vi "Print Report.vi"(0 "report in":refnum<class "NI_HTML.lvclass">, 5 "printer name (default)":string, 9 "number of copies (1)":i32=1, 11 "error in (no error)":errorcluster) -> (4 "report out":refnum<class "NI_HTML.lvclass">, 15 "error out":errorcluster)   [LabVIEW 2020, in "NI_HTML.lvclass"]
doc: "Prints a report to a designated printer or to the default printer on the computer."
uses:
  NI_HTML.lvclass
  e:/builds/penguin/labview/branches/2020/dev/dist/vi.lib/Utility/NIReport.llb/NI_report.lvclass
  NI_ReportGenerationCore.lvlib
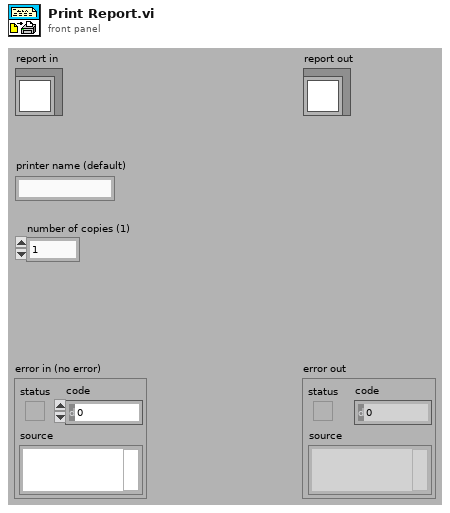
[diagram p1: front panel]
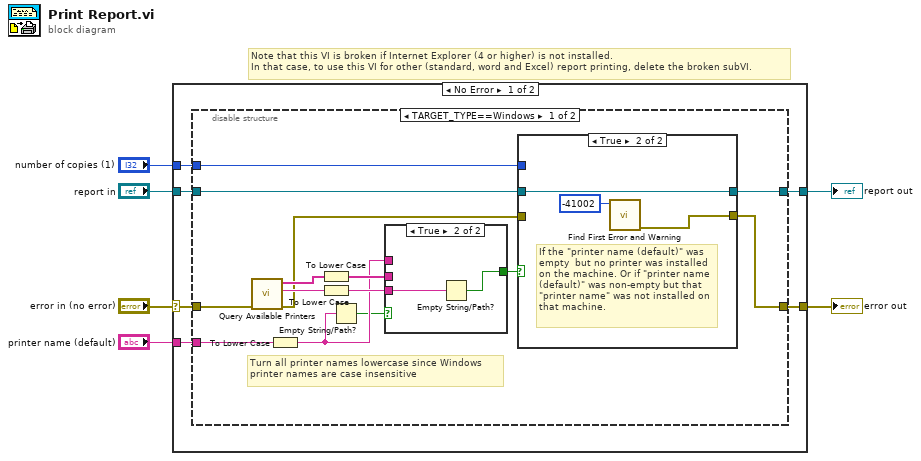
[diagram p0: block diagram]
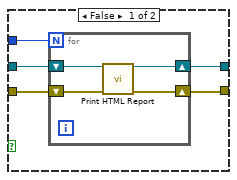
[diagram p2: hidden frame]
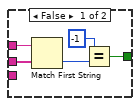
[diagram p3: hidden frame]
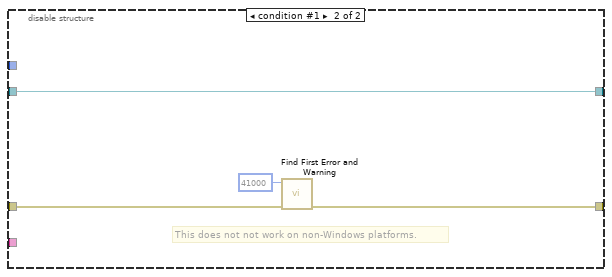
[diagram p4: hidden frame]
diagram:
  # "Note that this VI is broken if Internet Explorer (4 or higher) is not installed.\nIn that case, to use this VI for other (standard, word and Excel) report printing, delete the broken subVI."
  n1 = case shown="No Error" "error in (no error)" {
    selector: "error in (no error)" -> [w9 w51]
    tunnel: [w8 w51] -> w5
    tunnel: [w12 w50] -> w3
    tunnel: "report in" -> [w10 w50]
    tunnel: "printer name (default)" -> [w11 _]
    tunnel: "number of copies (1)" -> [w7 _]
    frame No Error {
      n2 = disable-structure shown="TARGET_TYPE==Windows" {
        disable-tunnel: [w18 w49] -> w12
        disable-tunnel: w11 -> [w17 _]
        disable-tunnel: w10 -> [w16 w49]
        disable-tunnel: w9 -> [w15 w47]
        disable-tunnel: [w14 w46] -> w8
        disable-tunnel: w7 -> [w13 _]
        frame condition #0 (active) {
          # "Turn all printer names lowercase since Windows\nprinter names are case insensitive"
          n3 = call "Query Available Printers.vi"("error in (no error)"=w15) -> ("error out"=w21:errorcluster, "default printer"=w23:string, "system configured printers"=w22:string[])  [unwired: 8 out]
          n4 = To Lower Case(string=w17) -> (all lower case string=w24:string)
          n5 = To Lower Case(string=w22) -> (all lower case string=w25:string[])
          n6 = To Lower Case(string=w23) -> (all lower case string=w26:string)
          n7 = Empty String/Path?(string/path=w24) -> (empty?=w19:bool)
          n8 = case shown="True" w19 {
            tunnel: w24 -> [w39 _]
            tunnel: [w40 w45] -> w20
            tunnel: w25 -> [w41 _]
            tunnel: w26 -> [_ w44]
            frame False {
              n9 = Match First String(2:w41, 3:w39) -> (0:w43:i32)  [unwired: 1 out]
              n10 = Equal?(x=-1 ("y"), y=w43) -> (x = y?=w40:bool)
            }
            frame True {
              n11 = Empty String/Path?(string/path=w44) -> (empty?=w45:bool)
            }
          }
          n12 = case shown="True" w20 {
            tunnel: w16 -> [w31 w36]
            tunnel: [w30 w36] -> w18
            tunnel: [w29 w38] -> w14
            tunnel: w21 -> [w28 _]
            tunnel: w13 -> [w27 _]
            frame False {
              n13 = for {
                N: w27 -> [_]
                shift-right: [w34] -> w30
                shift-left: w31 -> [w35]
                shift-right: [w33] -> w29
                shift-left: w28 -> [w32]
                n14 = call "Print HTML Report.vi"("report in"=w35, "error in (no error)"=w32) -> ("report out"=w34:refnum<class "NI_HTML.lvclass">, "error out"=w33:errorcluster)  [unwired: 12 out]
              }
            }
            frame True {
              # "If the \"printer name (default)\" was empty  but no printer was installed on the machine. Or if \"printer name (default)\" was non-empty but that \"printer name\" was not installed on that machine."
              n15 = call "Find First Error and Warning.vi"("error code"=-41002) -> ("error out"=w38:errorcluster)  [unwired: 1 in, 5 out]
            }
          }
        }
        frame condition #1 {
          # "This does not not work on non-Windows platforms."
          n16 = call "Find First Error and Warning.vi"("error in (no error)"=w47, "error code"=41000) -> ("error out"=w46:errorcluster)  [unwired: 4 in, 1 out]
        }
      }
    }
    frame Error {
    }
  }
  "error out" <- w5
  "report out" <- w3
